vi "SerialNew.vi"(8 "error in (no error)":errorcluster caption="错误输入（无错误）", 11 "serial 输入":refnum<class "serial.lvclass">) -> (0 "error out":errorcluster caption="错误输出", 2 "Serial I/O(记录)":refnum<visa-resource-name>, 3 "serial 输出":refnum<class "serial.lvclass">)   [LabVIEW 2019, in "serial.lvclass"]
uses:
  serial.lvclass
  serial.lvclass/serial.ctl
  <vilib>/Instr/_visa.llb/VISA Configure Serial Port (Instr).vi
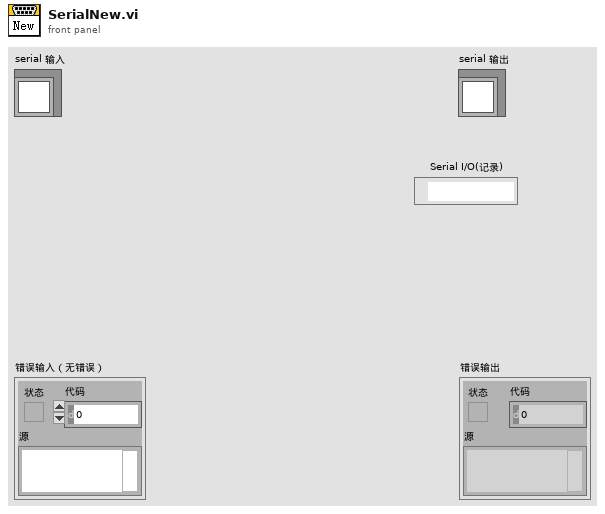
[diagram p1: front panel]
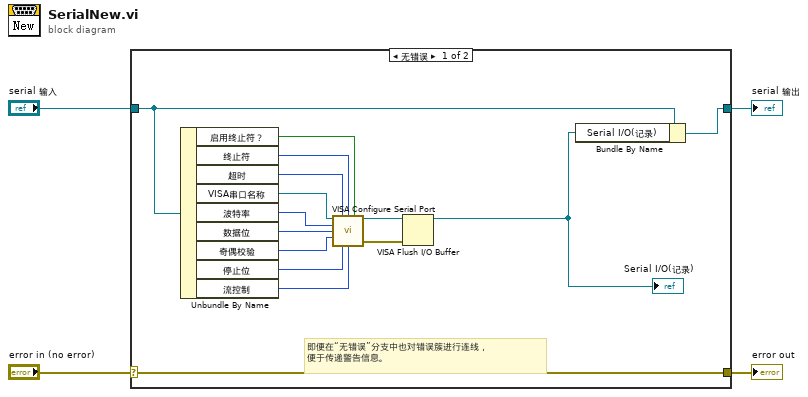
[diagram p0: block diagram]
diagram:
  n1 = case shown="无错误" "error in (no error)" {
    selector: "error in (no error)" -> [w19 w21]
    tunnel: [w19 w21] -> w3
    tunnel: [w5 w20] -> w1
    tunnel: "serial 输入" -> [w7 w20]
    frame No Error {
      # "即便在“无错误”分支中也对错误簇进行连线，\n便于传递警告信息。"
      n2 = Unbundle By Name(w7) -> ("启用终止符？"=w16:bool, "终止符"=w15:u8, "超时"=w14:u32, "VISA串口名称"=w13:refnum<visa-resource-name>, "波特率"=w12:u32, "数据位"=w11:u16, "奇偶校验"=w10:enum16{"None", "Odd", "Even", "Mark", "Space"}, "停止位"=w9:u16, "流控制"=w8:u16)
      n3 = call-poly "VISA Configure Serial Port"("VISA resource name"=w13, "timeout (10sec)"=w14, "termination char\n(0xA = '\\n' = LF)"=w15, "Enable Termination\nChar (T)"=w16, "baud rate (9600)"=w12, "data bits (8)"=w11, "parity (0:none)"=w10, "stop bits (10: 1 bit)"=w9, "flow control (0:none)"=w8) -> ("VISA resource name out"=w18:refnum<visa-resource-name>, "error out"=w17:errorcluster)  [unwired: 5 in]
      n4 = VISA Flush I/O Buffer(VISA resource name=w18, error in (no error)=w17) -> (VISA resource name out=w6:refnum<visa-resource-name>)  [unwired: 1 in, 1 out]
      "Serial I/O(记录)" <- w6
      n5 = Bundle By Name(cluster=w7, "Serial I/O(记录)"=w6) -> (w5:refnum<class "serial.lvclass">)
    }
    frame Error {
    }
  }
  "error out" <- w3
  "serial 输出" <- w1
